vi "BuildGetPacketParams.vi"(0 "DevType":T2(ring), 1 "Ch num":u8(ring) items=["Ch 1"], 2 "type":u32=1, 3 "Numeric":i32=4, 4 "UnitType":T1(ring)) -> (9 "Array":T3(array[cluster]))   [LabVIEW 2017]
panel:
  in  "Ch num 2":u8(ring) items=["Ch 1"]
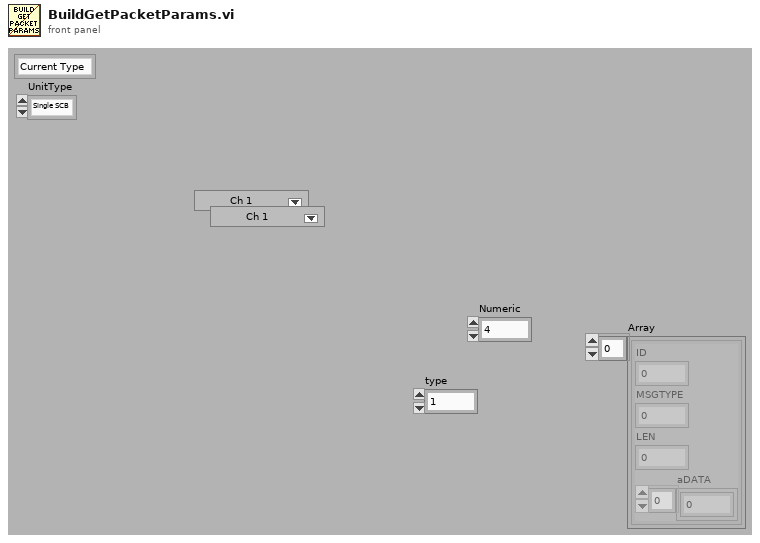
[diagram p1: front panel]
types:
  T1 = enum16{"Single SCB", "Power Rider", "Power Rider&Next10", "HATAL", "DAPH", "Indefinite", "Power Rider 12"}
  T2 = enum16{"Current Type", "Type 1", "Type 2", "Type 3", "Type 4", "Type 5", "Type 6", "Type 7", "Type 8", "Type 9", "Type 10"}
  T3 = cluster{"ID":u32, "MSGTYPE":u8, "LEN":u8, "aDATA":u8[]}[]
  T4 = cluster{"ID":u32, "MSGTYPE":u8, "LEN":u8, "aDATA":u8[]}
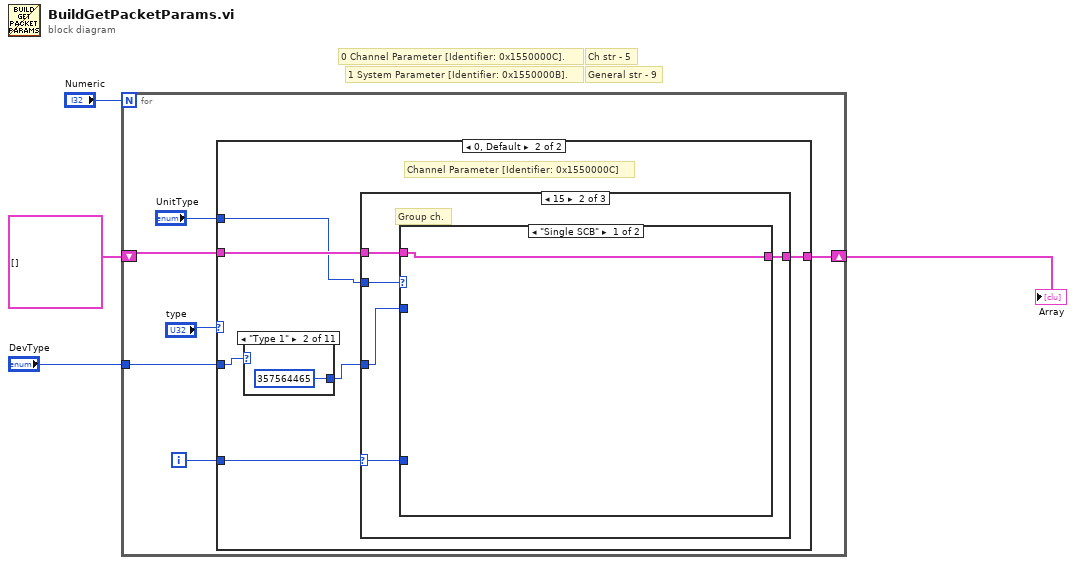
[diagram p0: block diagram]
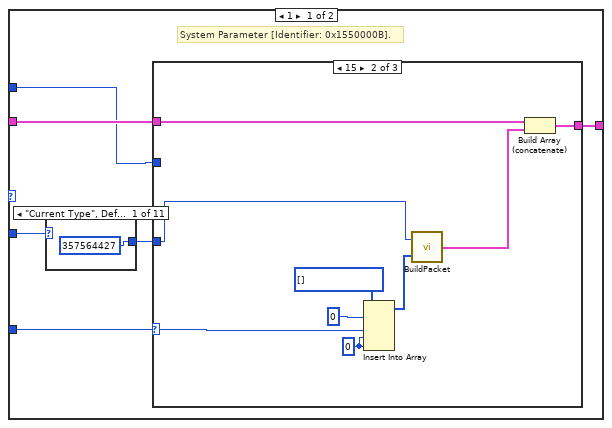
[diagram p2: hidden frame]
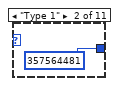
[diagram p3: hidden frame]
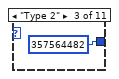
[diagram p4: hidden frame]
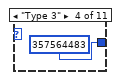
[diagram p5: hidden frame]
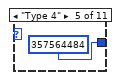
[diagram p6: hidden frame]
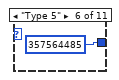
[diagram p7: hidden frame]
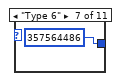
[diagram p8: hidden frame]
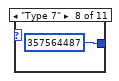
[diagram p9: hidden frame]
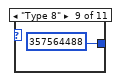
[diagram p10: hidden frame]
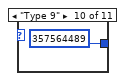
[diagram p11: hidden frame]
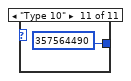
[diagram p12: hidden frame]
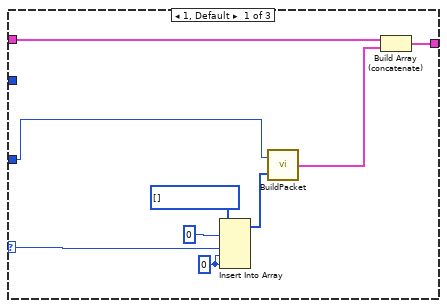
[diagram p13: hidden frame]
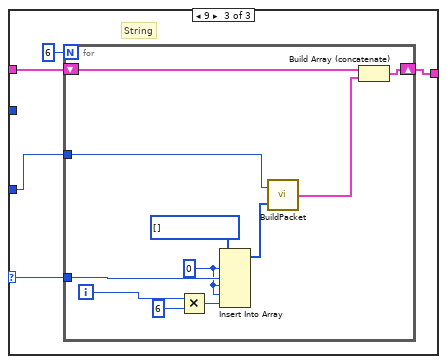
[diagram p14: hidden frame]
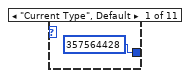
[diagram p15: hidden frame]
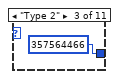
[diagram p16: hidden frame]
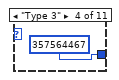
[diagram p17: hidden frame]
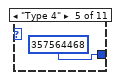
[diagram p18: hidden frame]
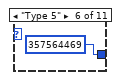
[diagram p19: hidden frame]
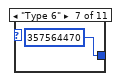
[diagram p20: hidden frame]
diagram:
  # "0 Channel Parameter [Identifier: 0x1550000C]."
  # "1 System Parameter [Identifier: 0x1550000B]."
  # "Ch str - 5"
  # "General str - 9"
  n1 = for {
    N: "Numeric" -> [_]
    shift-right: [w9] -> w2
    shift-left: T3 [] ("Array") -> [w10]
    tunnel: "DevType" -> [w6]
    i -> [w8]
    n2 = case shown="0, Default" "type" {
      tunnel: w10 -> [w16 w67]
      tunnel: [w15 w66] -> w9
      tunnel: w8 -> [w14 w65]
      tunnel: w6 -> [w13 w64]
      tunnel: "UnitType" -> [w11 w62]
      frame 1 {
        # "System Parameter [Identifier: 0x1550000B]."
        n3 = case shown="\"Current Type\", Default" w13 {
          tunnel: [u32 357564427 u32 357564481 u32 357564482 u32 357564483 u32 357564484 u32 357564485 u32 357564486 u32 357564487 u32 357564488 u32 357564489 u32 357564490] -> w12
          frame "Current Type", Default {
          }
          frame "Type 1" {
          }
          frame "Type 2" {
          }
          frame "Type 3" {
          }
          frame "Type 4" {
          }
          frame "Type 5" {
          }
          frame "Type 6" {
          }
          frame "Type 7" {
          }
          frame "Type 8" {
          }
          frame "Type 9" {
          }
          frame "Type 10" {
          }
        }
        n4 = case shown="15" w14 {
          selector: w14 -> [w33 w43 w49]
          tunnel: w16 -> [w36 w45 w50]
          tunnel: [w35 w44 w48] -> w15
          tunnel: w12 -> [w28 w42 w46]
          tunnel: w11 -> [_ _ _]
          frame 1, Default {
            w29 = u8 0 ("new element/subarray")
            n5 = Insert Into Array(array=u8[] [] ("Data 2"), index=0, new element #1=w33, new element #2=w29, new element #3=w29) -> (w30:u8[])
            n6 = call "BuildPacket.vi"("Data"=w30, "TxID"=w28) -> ("MsgTX 2"=w34:T4)
            n7 = Build Array (concatenate)(w36, w34) -> (w35:T3)
          }
          frame 15 {
            w37 = u8 0 ("new element/subarray")
            n8 = Insert Into Array(array=u8[] [] ("Data 2"), index=0, new element #1=w43, new element #2=w37, new element #3=w37) -> (w38:u8[])
            n9 = call "BuildPacket.vi"("Data"=w38, "TxID"=w42) -> ("MsgTX 2"=w41:T4)
            n10 = Build Array (concatenate)(w45, w41) -> (w44:T3)
          }
          frame 9 {
            # "String"
            n11 = for {
              N: 6 -> [_]
              tunnel: w49 -> [w59]
              shift-right: [w58] -> w48
              shift-left: w50 -> [w61]
              tunnel: w46 -> [w51]
              i -> [w54]
              w52 = 0 ("index")
              n12 = Multiply(x=w54, y=6) -> (x*y=w53:i32)
              n13 = Insert Into Array(array=u8[] [] ("Data 2"), index=w52, new element #1=w59, new element #2=w52, new element #3=w52, new element #4=w53) -> (w56:u8[])
              n14 = call "BuildPacket.vi"("Data"=w56, "TxID"=w51) -> ("MsgTX 2"=w60:T4)
              n15 = Build Array (concatenate)(w61, w60) -> (w58:T3)
            }
          }
        }
      }
      frame 0, Default {
        # "Channel Parameter [Identifier: 0x1550000C]"
        n16 = case shown="\"Type 1\"" w64 {
          tunnel: [u32 357564428 u32 357564465 u32 357564466 u32 357564467 u32 357564468 u32 357564469 u32 357564470 u32 357564471 u32 357564472 u32 357564473 u32 357564474] -> w63
          frame "Current Type", Default {
          }
          frame "Type 1" {
          }
          frame "Type 2" {
          }
          frame "Type 3" {
          }
          frame "Type 4" {
          }
          frame "Type 5" {
          }
          frame "Type 6" {
          }
          frame "Type 7" {
          }
          frame "Type 8" {
          }
          frame "Type 9" {
          }
          frame "Type 10" {
          }
        }
        n17 = case shown="15" w65 {
          selector: w65 -> [w85 w91 w108]
          tunnel: w67 -> [w88 w93 w109]
          tunnel: [w87 w92 w107] -> w66
          tunnel: w63 -> [w79 w90 w105]
          tunnel: w62 -> [_ w89 _]
          frame 1, Default {
            w80 = u8 0 ("new element/subarray")
            n18 = Insert Into Array(array=u8[] [] ("Data 2"), index=0, new element #1=w85, new element #2="Ch num", new element #3=w80, new element #4=w80) -> (w83:u8[])
            n19 = call "BuildPacket.vi"("Data"=w83, "TxID"=w79) -> ("MsgTX 2"=w86:T4)
            n20 = Build Array (concatenate)(w88, w86) -> (w87:T3)
          }
          frame 15 {
            # "Group ch."
            n21 = case shown="\"Single SCB\"" w89 {
              tunnel: w93 -> [w94 w104]
              tunnel: [w94 w103] -> w92
              tunnel: w91 -> [_ w101]
              tunnel: w90 -> [_ w95]
              frame "Single SCB" {
              }
              frame "Power Rider", Default {
                w96 = u8 0 ("new element/subarray")
                n22 = Insert Into Array(array=u8[] [] ("Data 2"), index=0, new element #1=w101, new element #2="Ch num 2", new element #3=w96, new element #4=w96) -> (w99:u8[])
                n23 = call "BuildPacket.vi"("Data"=w99, "TxID"=w95) -> ("MsgTX 2"=w102:T4)
                n24 = Build Array (concatenate)(w104, w102) -> (w103:T3)
              }
            }
          }
          frame 5 {
            # "String"
            n25 = for {
              N: 6 -> [_]
              tunnel: w108 -> [w120]
              shift-right: [w119] -> w107
              shift-left: w109 -> [w122]
              tunnel: w105 -> [w110]
              i -> [w114]
              n26 = local read "Ch num"() -> (w115:u8)
              n27 = Multiply(x=w114, y=6) -> (x*y=w112:i32)
              n28 = Insert Into Array(array=u8[] [] ("Data 2"), index=0, new element #1=w120, new element #2=w115, new element #3=u8 0 ("new element/subarray"), new element #4=w112) -> (w117:u8[])
              n29 = call "BuildPacket.vi"("Data"=w117, "TxID"=w110) -> ("MsgTX 2"=w121:T4)
              n30 = Build Array (concatenate)(w122, w121) -> (w119:T3)
            }
          }
        }
      }
    }
  }
  "Array" <- w2
